vi "Gabor Order Tracking Start-up.vi"() -> ()   [LabVIEW 2017]
doc: "This the VI that shows all toolkit features."
panel:
  out "left_top":bool
  out "selected item":string
  in  "STOP":bool
  in  "Select Demo":string(tree)="Order Analyzer"
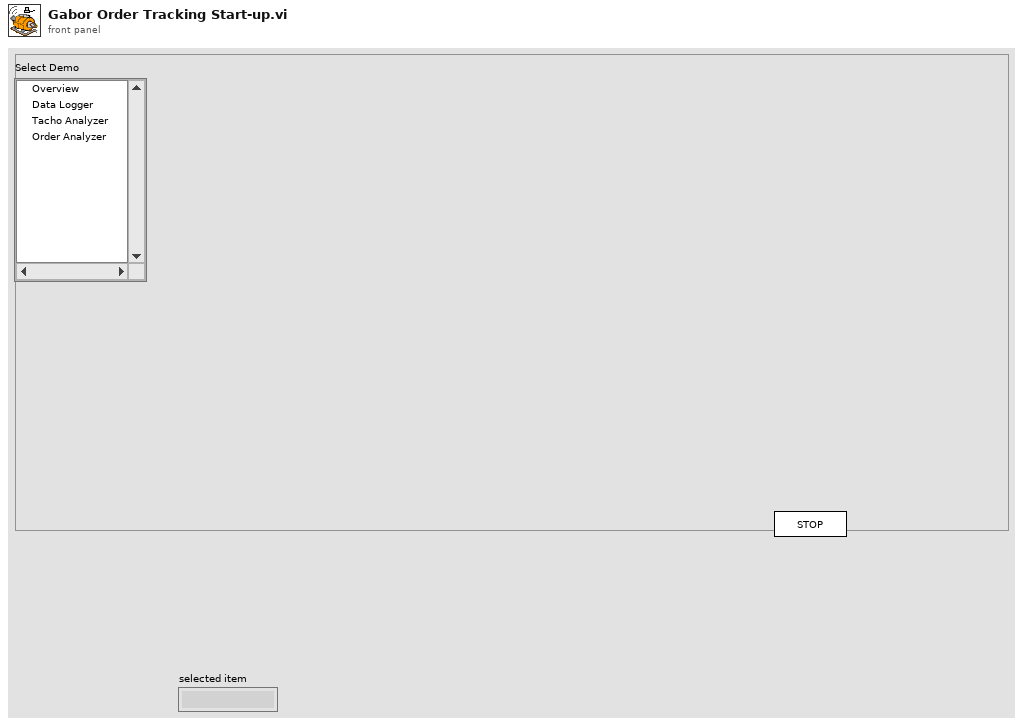
[diagram p1: front panel]
types:
  T1 = typedef "LVPositionTypeDef.ctl" = cluster{"Left":i32, "Top":i32}
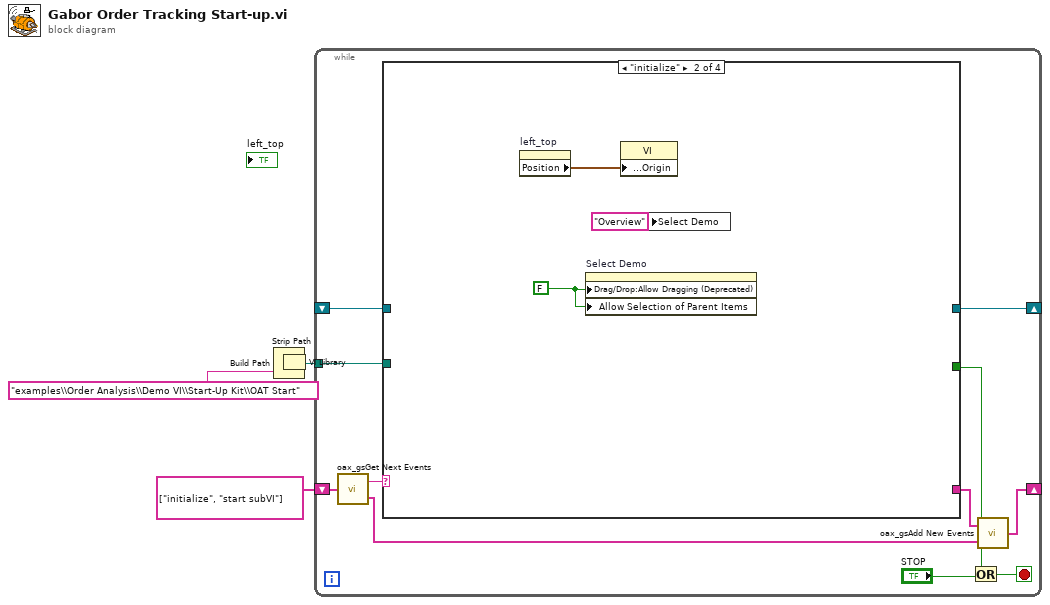
[diagram p0: block diagram]
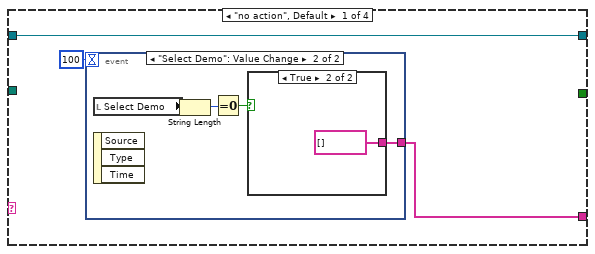
[diagram p2: hidden frame]
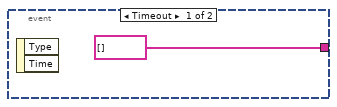
[diagram p3: hidden frame]
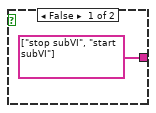
[diagram p4: hidden frame]
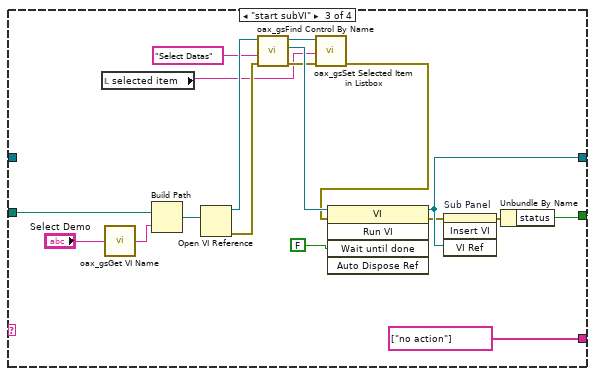
[diagram p5: hidden frame]
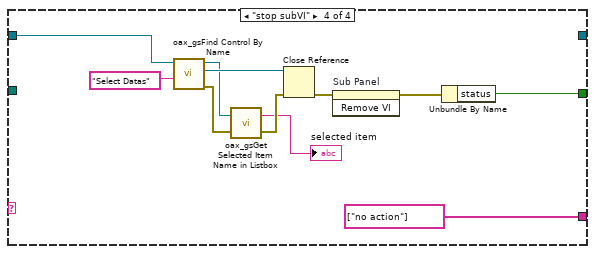
[diagram p6: hidden frame]
diagram:
  n1 = VI Library() -> (path=w4:path)
  n2 = Strip Path(path=w4) -> (stripped path=w5:path)  [unwired: 1 out]
  n3 = Build Path(base path=w5, name or relative path="examples\\Order Analysis\\Demo VI\\Start-Up Kit\\OAT Start") -> (appended path=w2:path)
  n4 = while {
    tunnel: w2 -> [w16]
    shift-right: [w15] -> _
    shift-left: _ -> [w14]
    shift-right: [w9] -> _
    shift-left: string[] ["initialize", "start subVI"] -> [w13]
    stop <- w6 stop-if-true
    n5 = call <vilib>:"oax_gsGet Next Events.vi"("event queue in"=w13) -> ("next event"=w12:string, "event queue out"=w11:string[])
    n6 = case shown="\"initialize\"" w12 {
      tunnel: w16 -> [_ _ w47 _]
      tunnel: [w19 _ w45 _] -> w15
      tunnel: w14 -> [w19 _ _ w54]
      tunnel: [_ _ w46 w58] -> w7
      tunnel: [w17 _ string[] ["no action"] string[] ["no action"]] -> w10
      frame "no action", Default {
        n7 = event shown="[1] \"Select Demo\": Value Change" {
          selector: _ -> [_ _]
          dyn-events: _ -> [_ _]
          timeout: 100 -> [_ _]
          tunnel: [string[] [] ("f") w24] -> w17
          event Timeout {
            n8 = event-data() -> ()  [unwired: 1 in, 2 out]
          }
          event "Select Demo": Value Change {
            n9 = local read "Select Demo"() -> (w22:string)
            n10 = event-data() -> ()  [unwired: 1 in, 3 out]
            n11 = String Length(string=w22) -> (length=w23:i32)
            n12 = Equal To 0?(x=w23) -> (x = 0?=w21:bool)
            n13 = case shown="True" w21 {
              tunnel: [string[] ["stop subVI", "start subVI"] string[] []] -> w24
              frame False {
              }
              frame True {
              }
            }
          }
        }
      }
      frame "initialize" {
        w28 = FALSE ("Allow Dragging")
        n14 = property on="left_top" class="Bool (strict)"() -> ("Position"=w27:T1)  [unwired: 2 in, 2 out]
        n15 = property on="Select Demo" class="Tree (strict)"("Drag/Drop:Allow Dragging (Deprecated)"=w28, "Allow Selection of Parent Items"=w28) -> ()  [unwired: 2 in, 2 out]
        n16 = property class="VI"("Front Panel Window:Origin"=w27) -> ()  [unwired: 2 in, 2 out]
        n17 = local write "Select Demo"("Overview" ("tree")) -> ()
      }
      frame "start subVI" {
        n18 = local read "selected item"() -> (w31:string)
        n19 = call <vilib>:"oax_gsGet VI Name.vi"("tree"="Select Demo") -> ("vi name"=w42:string)
        n20 = Build Path(base path=w47, name or relative path=w42) -> (appended path=w41:path)
        n21 = Open VI Reference(vi path=w41) -> (vi reference=w36:refnum<vi>, error out=w37:errorcluster)  [unwired: 5 in]
        n22 = call <vilib>:"oax_gsFind Control By Name.vi"("error in (no error)"=w37, "control name"="Select Datas", "vi refnum in"=w36) -> ("error out"=w32:errorcluster, "vi refnum out"=w35:refnum<vi>, "control refnum"=w33:refnum<vi>)  [unwired: 6 in]
        n23 = call <vilib>:"oax_gsSet Selected Item in Listbox.vi"("error in (no error)"=w32, "item name"=w31, "control refnum"=w33) -> ("error out"=w30:errorcluster)  [unwired: 6 in, 2 out]
        n24 = invoke class="VI" method="Run VI"(reference=w35, error in=w30, "Wait until done"=FALSE) -> (reference out=w45:refnum<vi>, error out=w39:errorcluster)  [unwired: 2 in, 3 out]
        n25 = invoke on="Sub Panel" class="SubPanel" method="Insert VI"(error in=w39, "VI Ref"=w45) -> (error out=w38:errorcluster)  [unwired: 2 in, 3 out]
        n26 = Unbundle By Name(w38) -> ("status"=w46:bool)
      }
      frame "stop subVI" {
        n27 = call <vilib>:"oax_gsFind Control By Name.vi"("control name"="Select Datas", "vi refnum in"=w54) -> ("error out"=w50:errorcluster, "vi refnum out"=w53:refnum<vi>, "control refnum"=w51:refnum<vi>)  [unwired: 7 in]
        n28 = call <vilib>:"oax_gsGet Selected Item Name in Listbox.vi"("error in (no error)"=w50, "ctrl reference"=w51) -> ("error out"=w49:errorcluster, "selected item"=→"selected item":string)
        n29 = Close Reference(reference=w53, error in (no error)=w49) -> (error out=w56:errorcluster)
        n30 = invoke on="Sub Panel" class="SubPanel" method="Remove VI"(error in=w56) -> (error out=w55:errorcluster)  [unwired: 2 in, 2 out]
        n31 = Unbundle By Name(w55) -> ("status"=w58:bool)
      }
    }
    n32 = Or(x=w7, y="STOP") -> (x .or. y?=w6:bool)
    n33 = call <vilib>:"oax_gsAdd New Events.vi"("event in"=w11, "new events"=w10) -> ("event out"=w9:string[])
  }
